vi "Set Window State.vi"(8 "error in (no error)":errorcluster, 10 "State":T1(ring), 11 "Actor in":refnum<class "Actor.lvclass">) -> (0 "error out":errorcluster)   [LabVIEW 2020, in "RTAF.lvlib" / "Actor.lvclass"]
uses:
  Actor.lvclass
  Actor.lvclass/Actor.ctl
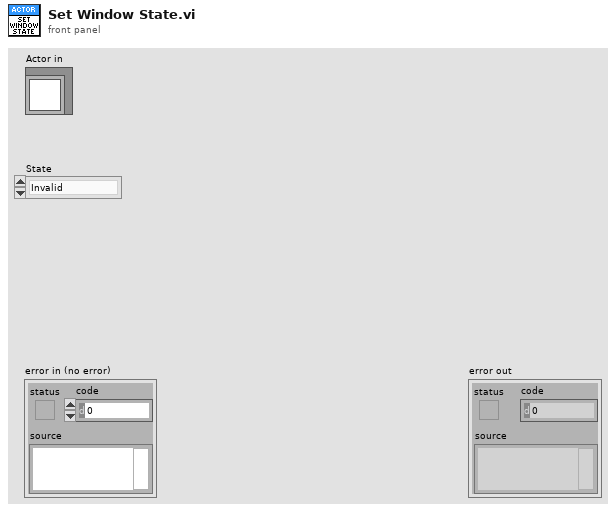
[diagram p1: front panel]
types:
  T1 = enum32{"Invalid", "Standard", "Closed", "Hidden", "Minimized", "Maximized"}
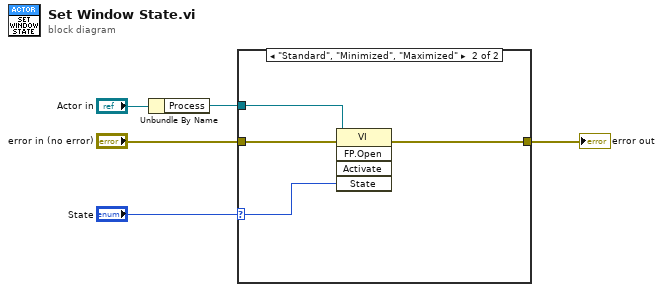
[diagram p0: block diagram]
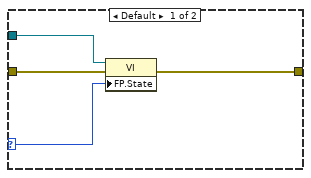
[diagram p2: hidden frame]
diagram:
  n1 = Unbundle By Name("Actor in") -> ("Process"=w3:refnum<vi>)
  n2 = case shown="\"Standard\", \"Minimized\", \"Maximized\"" "State" {
    selector: "State" -> [w6 w11]
    tunnel: "error in (no error)" -> [w8 w13]
    tunnel: w3 -> [w9 w12]
    tunnel: [w7 w10] -> w2
    frame Default {
      n3 = property class="VI"(reference=w9, error in=w8, "FP.State"=w6) -> (error out=w7:errorcluster)  [unwired: 1 out]
    }
    frame "Standard", "Minimized", "Maximized" {
      n4 = invoke class="VI" method="FP.Open"(reference=w12, error in=w13, "State"=w11) -> (error out=w10:errorcluster)  [unwired: 2 in, 4 out]
    }
  }
  "error out" <- w2
